vi "Destroy Messaging Network.vi"(8 "error in (no error)":errorcluster, 11 "msg cluster":T1) -> (0 "error out":errorcluster)   [LabVIEW 2020]
uses:
  Messaging Cluster.ctl
  Hardware/Sensors/Cameras/Camera.lvclass
  Hardware/Sensors/Force Sensors/Force Sensor.lvclass
  Hardware/Actuators/Servos/Servo.lvclass
  Hardware/Actuators/Switches/Switch.lvclass
  Controller Loop/Message and Data.ctl
  Inflation Test/Parameter Class/IA Test Parameters.lvclass
  Controllers/Controller.lvclass
  File Interfacing/Filename Structure.ctl
  GUI/Main GUI Loop/Handler.ctl
  Inflation Test/Result Handling/Inflation Test Numeric Results.ctl
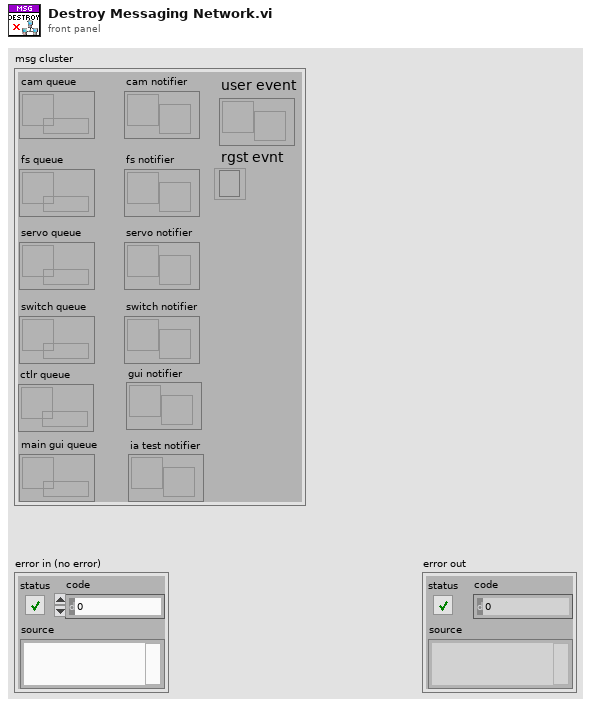
[diagram p1: front panel]
types:
  T1 = typedef "Messaging Cluster.ctl" = cluster{"cam queue":refnum<queue>, "fs queue":refnum<queue>, "servo queue":refnum<queue>, "switch queue":refnum<queue>, "switch notifier":refnum<notifier>, "servo notifier":refnum<notifier>, "fs notifier":refnum<notifier>, "cam notifier":refnum<notifier>, "rgst evnt":refnum<event-registration>, "user event":refnum<user-event>, "ctlr queue":refnum<queue>, "main gui queue":refnum<queue>, "gui notifier":refnum<notifier>, "ia test notifier":refnum<notifier>}
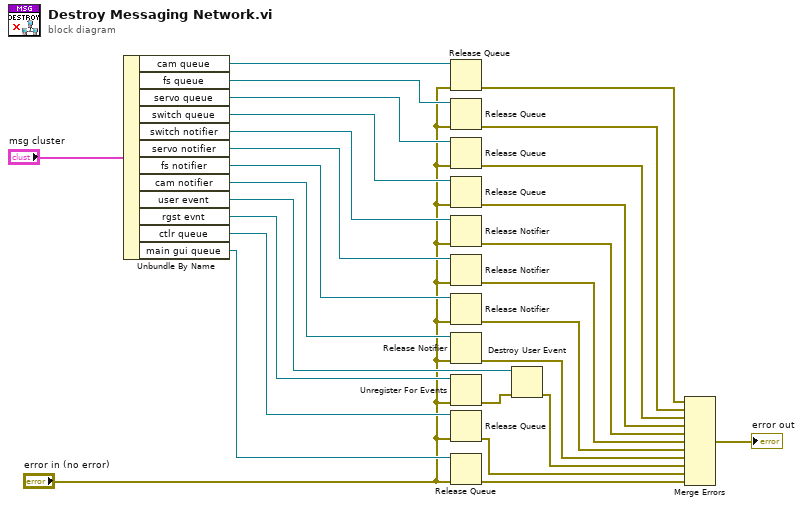
[diagram p0: block diagram]
diagram:
  n1 = Unbundle By Name("msg cluster") -> ("cam queue"=w26:refnum<queue>, "fs queue"=w25:refnum<queue>, "servo queue"=w24:refnum<queue>, "switch queue"=w23:refnum<queue>, "switch notifier"=w22:refnum<notifier>, "servo notifier"=w21:refnum<notifier>, "fs notifier"=w20:refnum<notifier>, "cam notifier"=w19:refnum<notifier>, "user event"=w16:refnum<user-event>, "rgst evnt"=w17:refnum<event-registration>, "ctlr queue"=w15:refnum<queue>, "main gui queue"=w14:refnum<queue>)
  n2 = Release Queue(queue=w26, error in (no error)="error in (no error)") -> (error out=w2:errorcluster)  [unwired: 1 in, 2 out]
  n3 = Release Queue(queue=w25, error in (no error)="error in (no error)") -> (error out=w3:errorcluster)  [unwired: 1 in, 2 out]
  n4 = Release Queue(queue=w24, error in (no error)="error in (no error)") -> (error out=w4:errorcluster)  [unwired: 1 in, 2 out]
  n5 = Release Queue(queue=w23, error in (no error)="error in (no error)") -> (error out=w5:errorcluster)  [unwired: 1 in, 2 out]
  n6 = Release Notifier(notifier=w22, error in (no error)="error in (no error)") -> (error out=w6:errorcluster)  [unwired: 1 in, 2 out]
  n7 = Release Notifier(notifier=w21, error in (no error)="error in (no error)") -> (error out=w7:errorcluster)  [unwired: 1 in, 2 out]
  n8 = Release Notifier(notifier=w20, error in (no error)="error in (no error)") -> (error out=w8:errorcluster)  [unwired: 1 in, 2 out]
  n9 = Release Notifier(notifier=w19, error in (no error)="error in (no error)") -> (error out=w9:errorcluster)  [unwired: 1 in, 2 out]
  n10 = Unregister For Events(event registration refnum=w17, error in="error in (no error)") -> (error out=w18:errorcluster)
  n11 = Release Queue(queue=w15, error in (no error)="error in (no error)") -> (error out=w11:errorcluster)  [unwired: 1 in, 2 out]
  n12 = Release Queue(queue=w14, error in (no error)="error in (no error)") -> (error out=w12:errorcluster)  [unwired: 1 in, 2 out]
  n13 = Destroy User Event(user event=w16, error in=w18) -> (error out=w10:errorcluster)
  n14 = Merge Errors(w2, w3, w4, w5, w6, w7, w8, w9, w10, w11, w12) -> (→"error out":errorcluster)
